vi "InitScan.vi"(8 "error in (no error)":errorcluster, 10 "event data":T1, 11 "SPIController in":refnum<class "SPIController.lvclass">) -> (0 "error out":errorcluster, 3 "SPIController out":refnum<class "SPIController.lvclass">)   [LabVIEW 2023, in "SPIController.lvlib" / "SPIController.lvclass"]
uses:
  SPIController.lvclass
  TranslationStage_UI/Arduino_Stepper_UI/Scan_Data_For_Controller.ctl
  SPIController.lvclass/SPIController.ctl
  typedefs/typedefs.lvlib
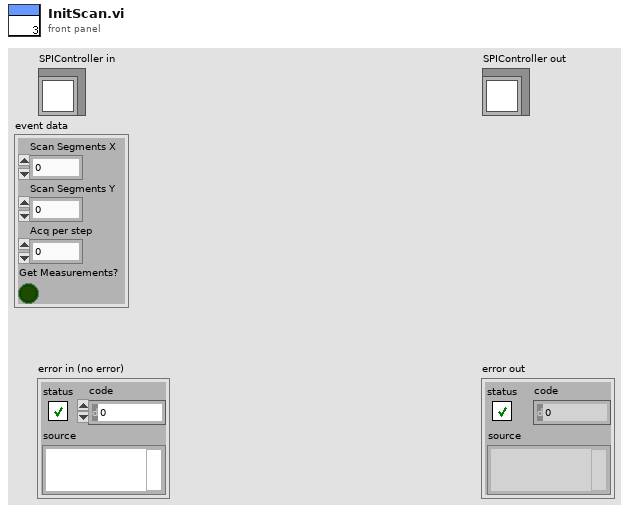
[diagram p1: front panel]
types:
  T1 = typedef "typedefs.lvlib/Scan_Data_For_Controller.ctl" = cluster{"Scan Segments X":u32, "Scan Segments Y":u32, "Acq per step":u8, "Get Measurements?":bool}
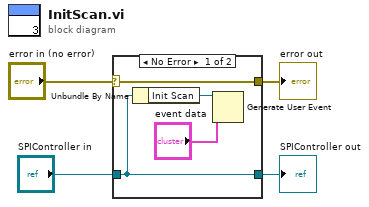
[diagram p0: block diagram]
diagram:
  n1 = case shown="No Error" "error in (no error)" {
    selector: "error in (no error)" -> [w8 w10]
    tunnel: [w8 w10] -> w3
    tunnel: [w7 w9] -> w1
    tunnel: "SPIController in" -> [w7 w9]
    frame No Error {
      n2 = Unbundle By Name(w7) -> ("Init Scan"=w6:refnum<user-event>)
      n3 = Generate User Event(user event=w6, event data cluster="event data") -> ()  [unwired: 2 in, 2 out]
    }
    frame Error {
    }
  }
  "error out" <- w3
  "SPIController out" <- w1
